vi "FTW-Actor-LocalMessage-Send-Lossy.vi"(0 "FTW-ActorInstance In":refnum<class "FTW-ActorInstance.lvclass">, 1 "FTW Message":refnum<class "FTW-Message.lvclass">, 5 "Message Header":string, 7 "Message Body":string, 11 "error in":errorcluster) -> (15 "error out":errorcluster)   [LabVIEW 2013, in "FTW-ActorInstance.lvclass"]
uses:
  FTW-ActorInstance.lvclass
  Message/Base/FTW-Message.lvclass
  Message/Lossy/FTW-Message-Lossy.lvclass
  FTW-ActorInstance.lvclass/FTW-ActorInstance.ctl
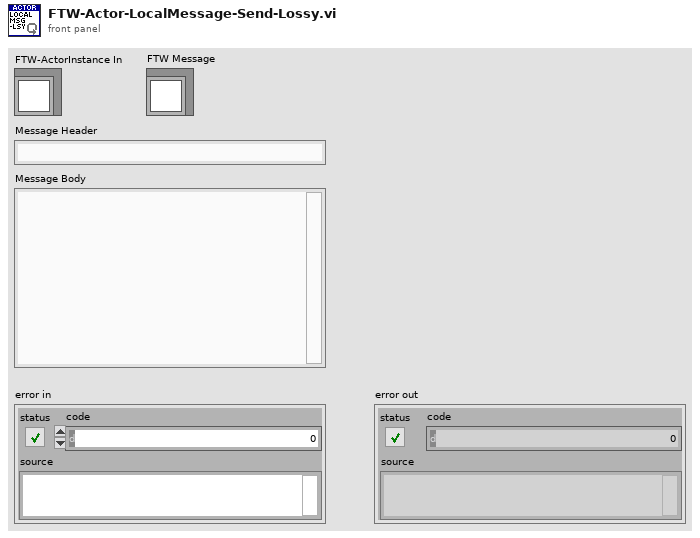
[diagram p1: front panel]
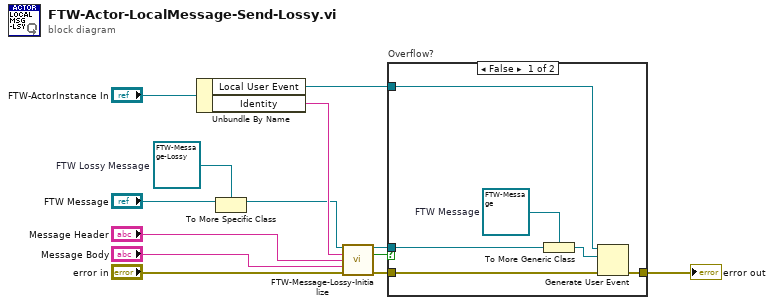
[diagram p0: block diagram]
diagram:
  w1 = refnum<class "FTW-Message-Lossy.lvclass"> refnum  # FTW Lossy Message
  n1 = Unbundle By Name("FTW-ActorInstance In") -> ("Local User Event"=w5:refnum<user-event>, "Identity"=w4:string)
  n2 = To More Specific Class(target class=w1, reference="FTW Message") -> (specific class reference=w2:refnum<class "FTW-Message-Lossy.lvclass">)  [unwired: 1 in, 1 out]
  n3 = call-dynamic "FTW-Message-Lossy-Initialize.vi"("FTW-Message-Lossy In"=w2, "Sender Identity"=w4, "Message Header"="Message Header", "Message Body"="Message Body", "error in"="error in") -> ("FTW-Message-Lossy Out"=w6:refnum<class "FTW-Message-Lossy.lvclass">, "overflow?"=w3:bool, "error out"=w7:errorcluster)  [unwired: 8 in]
  n4 = case "Overflow?" shown="False" w3 {
    tunnel: w7 -> [w18 w20]
    tunnel: w6 -> [w17 _]
    tunnel: [w16 w20] -> w11
    tunnel: w5 -> [w14 _]
    frame False {
      w15 = refnum<class "FTW-Message.lvclass"> refnum  # FTW Message
      n5 = To More Generic Class(target class=w15, reference=w17) -> (generic class reference=w19:refnum<class "FTW-Message.lvclass">)
      n6 = Generate User Event(user event=w14, event data cluster=w19, error in=w18) -> (error out=w16:errorcluster)  [unwired: 1 in, 1 out]
    }
    frame True {
      # "event handler has notifications\nfor all current messages\n\ndon't send any more UEs"
    }
  }
  "error out" <- w11
